vi "Set Default Grid Sizes.vi"(8 "error in (no error)":errorcluster, 11 "VI Ref":refnum<vi>) -> (0 "error out":errorcluster, 2 "Save?":bool, 3 "VI Ref out":refnum<vi>)   [LabVIEW 2020, in "Code Cleanup.lvlib"]
uses:
  Code Cleanup.lvlib
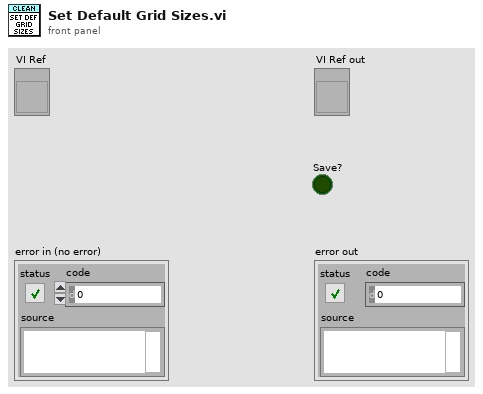
[diagram p1: front panel]
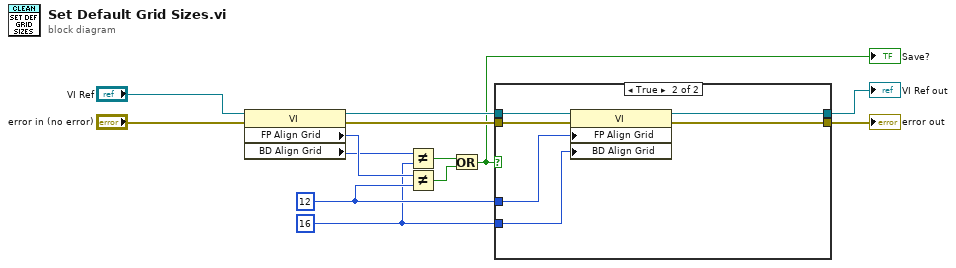
[diagram p0: block diagram]
diagram:
  w4 = 16 ("y")
  w5 = 12 ("y")
  n1 = property class="VI"(reference="VI Ref", error in="error in (no error)") -> (reference out=w6:refnum<vi>, error out=w7:errorcluster, "FP Align Grid"=w11:i32, "BD Align Grid"=w8:i32)
  n2 = Not Equal?(x=w8, y=w4) -> (x != y?=w10:bool)
  n3 = Not Equal?(x=w11, y=w5) -> (x != y?=w9:bool)
  n4 = Or(x=w10, y=w9) -> (x .or. y?=w2:bool)
  "Save?" <- w2
  n5 = case shown="True" w2 {
    tunnel: w7 -> [w15 w20]
    tunnel: [w15 w19] -> w12
    tunnel: [w14 w18] -> w1
    tunnel: w6 -> [w14 w21]
    tunnel: w5 -> [_ w16]
    tunnel: w4 -> [_ w17]
    frame False {
    }
    frame True {
      n6 = property class="VI"(reference=w21, error in=w20, "FP Align Grid"=w16, "BD Align Grid"=w17) -> (reference out=w18:refnum<vi>, error out=w19:errorcluster)
    }
  }
  "error out" <- w12
  "VI Ref out" <- w1
